vi "Untitled 4.vi"() -> ()   [LabVIEW 2017]
panel:
  out "date/time string":string
  out "error out 2":errorcluster
  out "Timestamp 2":timestamp
  out "*(type *) &x":string
  out "Timestamp":timestamp
  in  "error in":errorcluster
  out "error out":errorcluster
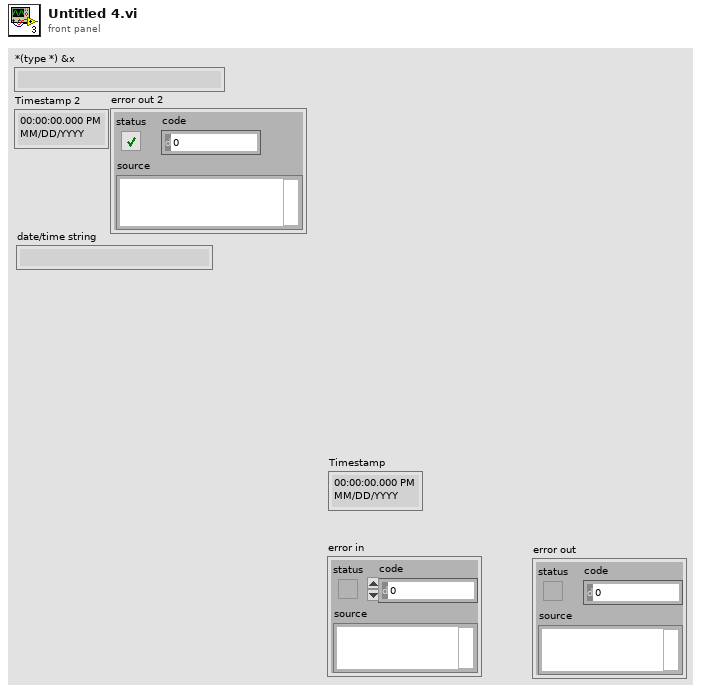
[diagram p1: front panel]
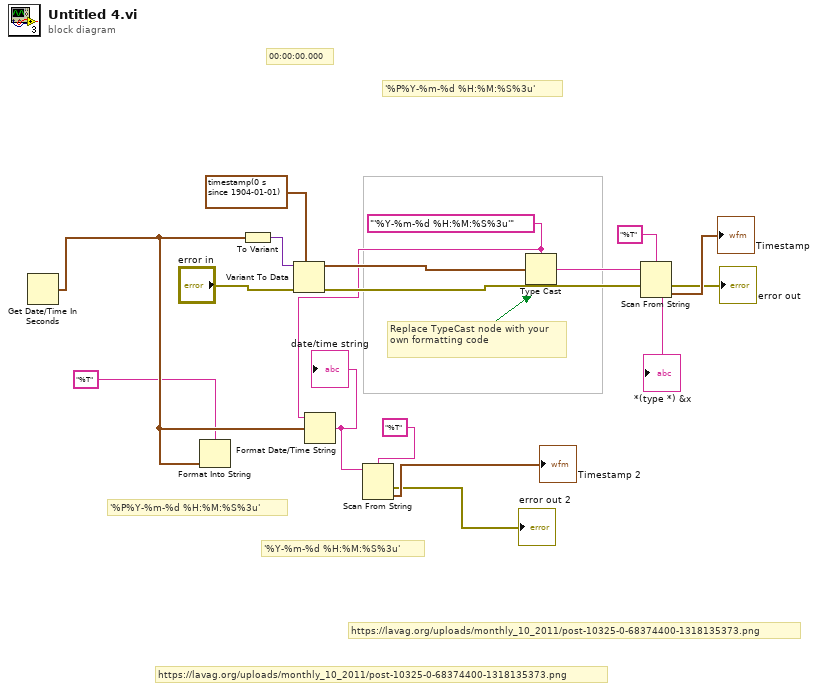
[diagram p0: block diagram]
diagram:
  w8 = "'%Y-%m-%d %H:%M:%S%3u'" ("type")
  # "'%P%Y-%m-%d %H:%M:%S%3u'"
  # "'%P%Y-%m-%d %H:%M:%S%3u'"
  # "https://lavag.org/uploads/monthly_10_2011/post-10325-0-68374400-1318135373.png"
  # "https://lavag.org/uploads/monthly_10_2011/post-10325-0-68374400-1318135373.png"
  # "'%Y-%m-%d %H:%M:%S%3u'"
  # "00:00:00.000"
  # "Replace TypeCast node with your own formatting code"
  n1 = Get Date/Time In Seconds() -> (seconds since 1Jan1904=w4:timestamp)
  n2 = Format Into String(format string="%T", w4) -> ()  [unwired: 2 in, 2 out]
  n3 = To Variant(anything=w4) -> (Variant=w14:variant)
  n4 = Variant To Data(error in="error in", type=timestamp(0 s since 1904-01-01) ("time stamp"), Variant=w14) -> (data=w12:timestamp, error out=w11:errorcluster)
  n5 = Format Date/Time String(time format string (%c)=w8, seconds (now)=w4) -> (date/time string=w1:string)  [unwired: 1 in]
  "date/time string" <- w1
  n6 = Scan From String(format string="%T", input string=w1) -> (error out=→"error out 2":errorcluster, output 1=→"Timestamp 2":timestamp)  [unwired: 3 in, 2 out]
  n7 = Type Cast(type=w8, x=w12) -> (*(type *) &x=w10:string)
  "*(type *) &x" <- w10
  n8 = Scan From String(format string="%T", input string=w10, error in=w11) -> (error out=→"error out":errorcluster, output 1=→"Timestamp":timestamp)  [unwired: 2 in, 2 out]
